vi "add new label.vi"(8 "error in (no error)":errorcluster, 9 "VI controls":refnum<vi>[](array[refnum]), 10 "all Label text":string[](array[string]), 11 "Language Data in":T2) -> (0 "error out":errorcluster, 3 "Language Data out":T2)   [LabVIEW 2015, in "AguaClara Library.lvlib"]
uses:
  AguaClara Library.lvlib
  language cmd.ctl
  Variable cluster.ctl
panel:
  in  "language cmd":T1
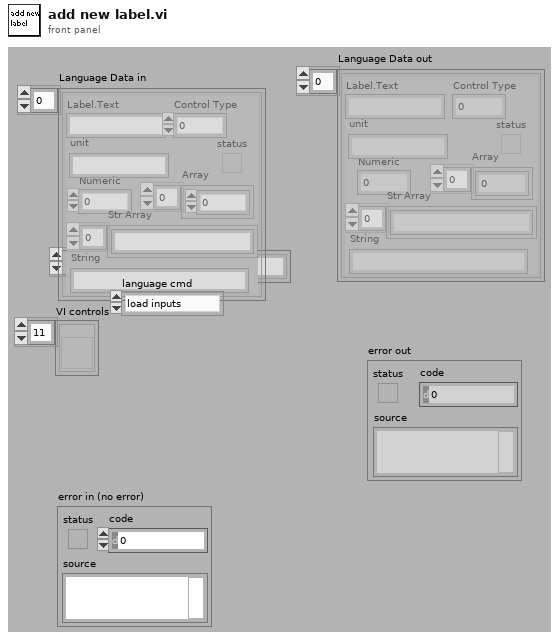
[diagram p1: front panel]
types:
  T1 = typedef "AguaClara Library.lvlib/language cmd.ctl" = enum16{"load inputs", "choose language", "translate", "load storage variable from file"}
  T2 = typedef "Variable cluster.ctl" = cluster{"Label.Text":string, "Control Type":u32, "Numeric":dbl, "Array":dbl[], "status":bool, "Str Array":string[], "String":string, "unit":string}[]
  T3 = cluster{"Label.Text":string, "Control Type":u32, "Numeric":dbl, "Array":dbl[], "status":bool, "Str Array":string[], "String":string, "unit":string}
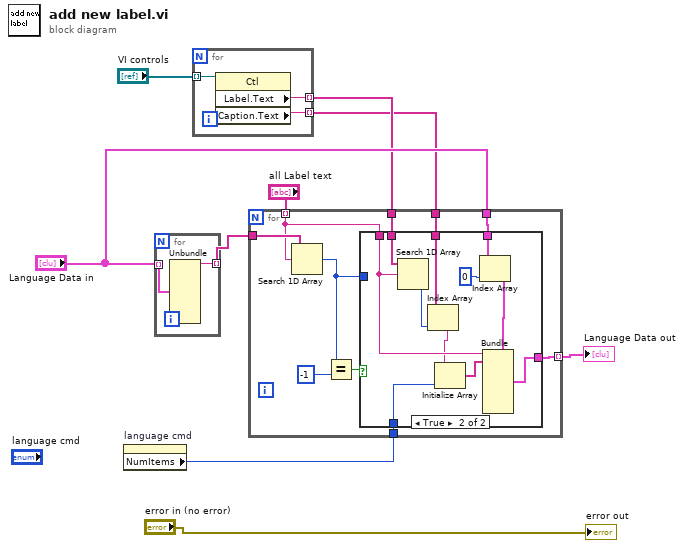
[diagram p0: block diagram]
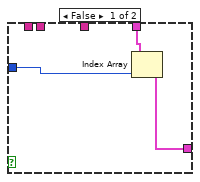
[diagram p2: hidden frame]
diagram:
  n1 = property on="language cmd" class="Enum (strict)"() -> ("NumItems"=w1:u32)  [unwired: 2 in, 2 out]
  n2 = for {
    tunnel: "Language Data in" -> [w11] mode=indexing
    tunnel: [w10] -> w9 mode=indexing
    n3 = Unbundle(w11) -> ("Label.Text"=w10:string)  [unwired: 7 out]
  }
  n4 = for {
    tunnel: "VI controls" -> [w14] mode=indexing
    tunnel: [w13] -> w3 mode=indexing
    tunnel: [w12] -> w2 mode=indexing
    n5 = property class="Ctl"(reference=w14) -> ("Label.Text"=w13:string, "Caption.Text"=w12:string)  [unwired: 1 in, 2 out]
  }
  n6 = for {
    tunnel: w9 -> [w24]
    tunnel: "all Label text" -> [w22] mode=indexing
    tunnel: "Language Data in" -> [w19]
    tunnel: [w18] -> w5 mode=indexing
    tunnel: w3 -> [w17]
    tunnel: w2 -> [w16]
    tunnel: w1 -> [w15]
    n7 = Search 1D Array(1D array=w24, element=w22) -> (index of element=w20:i32)  [unwired: 1 in]
    n8 = Equal?(x=w20, y=-1) -> (x = y?=w21:bool)
    n9 = case shown="True" w21 {
      tunnel: w22 -> [_ w33]
      tunnel: w20 -> [w27 _]
      tunnel: w19 -> [w26 w37]
      tunnel: [w25 w38] -> w18
      tunnel: w17 -> [_ w34]
      tunnel: w16 -> [_ w31]
      tunnel: w15 -> [_ w30]
      frame False {
        n10 = Index Array(array=w26, index=w27) -> (element=w25:T3)
      }
      frame True {
        n11 = Search 1D Array(1D array=w34, element=w33) -> (index of element=w32:i32)  [unwired: 1 in]
        n12 = Index Array(array=w31, index=w32) -> (element=w29:string)
        n13 = Initialize Array(w29, w30) -> (w28:string[])
        n14 = Index Array(array=w37, index=0) -> (element=w35:T3)
        n15 = Bundle(cluster=w35, "Label.Text"=w33, "Control Type"=w28) -> (w38:T3)  [unwired: 6 in]
      }
    }
  }
  "Language Data out" <- w5
  "error out" <- "error in (no error)"
